vi "HEWH Determine Intellifaucet Setting.vi"(8 "Error In":errorcluster, 10 "GPM Target":dbl, 11 "Calc and Calibration":T1) -> (0 "Error Out":errorcluster, 3 "Valve % Open":dbl)   [LabVIEW 2023]
uses:
  Type Definitions/HEWH Calc and Calibration.ctl
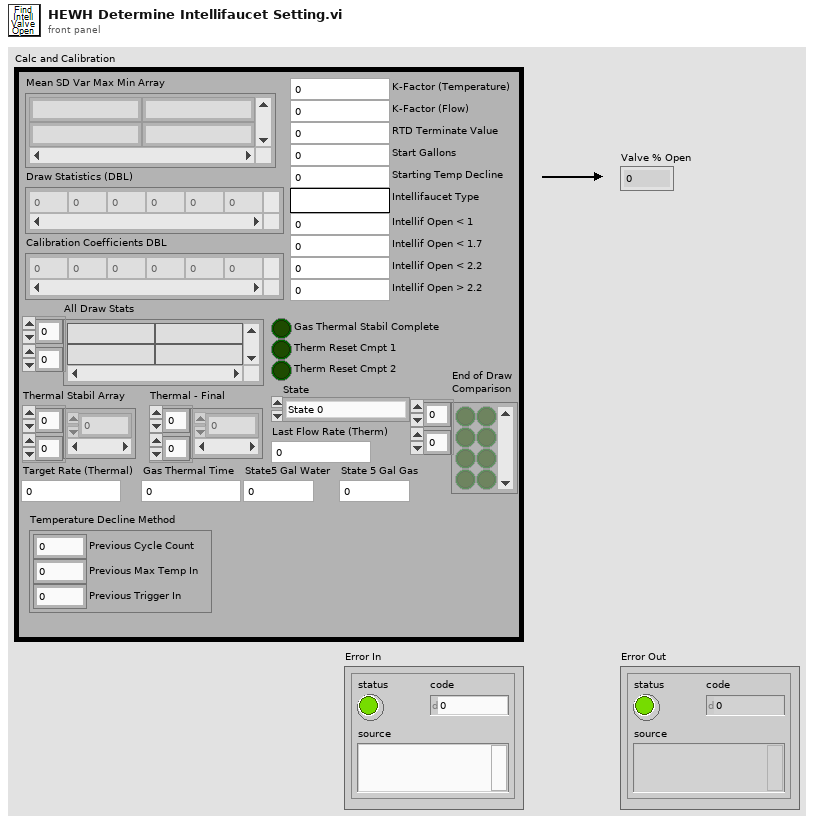
[diagram p1: front panel]
types:
  T1 = typedef "HEWH Calc and Calibration.ctl" = cluster{"Mean SD Var Max Min Array":string[][], "Draw Statistics (DBL)":dbl[][], "Calibration Coefficients DBL":dbl[][], "Start Gallons":dbl, "Starting Temp Decline":dbl, "K-Factor (Temperature)":dbl, "All Draw Stats":string[][], "RTD Terminate Value":dbl, "K-Factor (Flow)":dbl, "Intellifaucet Type":string, "Thermal Stabil Array":dbl[][], "Gas Thermal Stabil Complete":bool, "Therm Reset Cmpt 1":bool, "Therm Reset Cmpt 2":bool, "Last Flow Rate (Therm)":dbl, "State":enum16{"State 0", "State 1", "State 2", "State 3", "State 4", "State 5", "State 6"}, "Gas Thermal Time":dbl, "Target Rate (Thermal)":dbl, "Thermal - Final":dbl[][], "State5 Gal Water":dbl, "State 5 Gal Gas":dbl, "Intellif Open < 1":dbl, "Intellif Open < 1.7":dbl, "Intellif Open < 2.2":dbl, "Intellif Open > 2.2":dbl, "End of Draw\nComparison":bool[][], "Temperature Decline Method":cluster{"Previous Cycle Count":i32, "Previous Max Temp In":dbl, "Previous Trigger In":u8}}
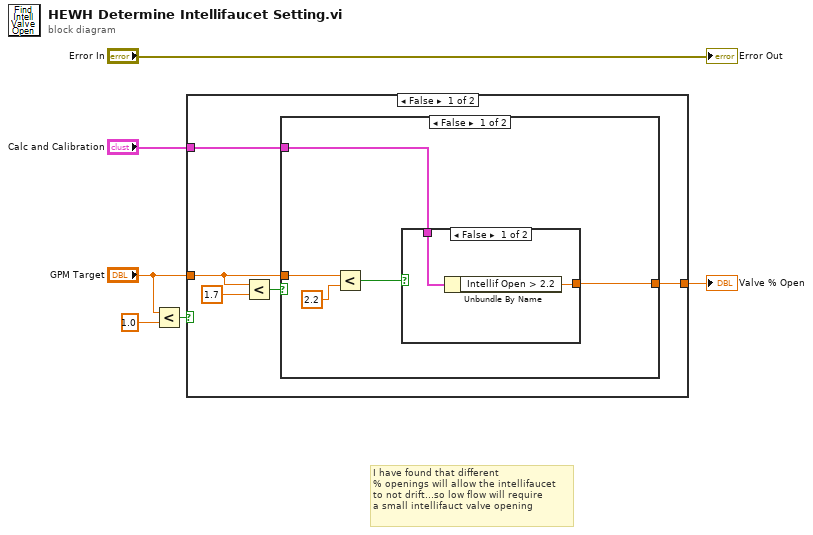
[diagram p0: block diagram]
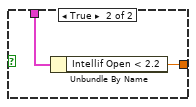
[diagram p2: hidden frame]
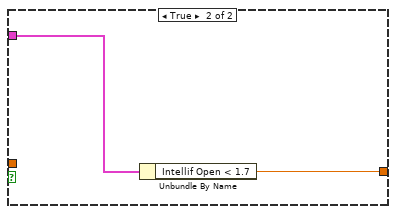
[diagram p3: hidden frame]
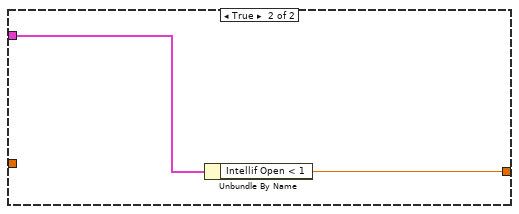
[diagram p4: hidden frame]
diagram:
  # "I have found that different\n% openings will allow the intellifaucet\nto not drift...so low flow will require\na small intellifauct valve opening"
  n1 = Less?(x="GPM Target", y=1.0) -> (x < y?=w4:bool)
  n2 = case shown="False" w4 {
    tunnel: "GPM Target" -> [w11 _]
    tunnel: [w8 w23] -> w6
    tunnel: "Calc and Calibration" -> [w7 w24]
    frame False {
      n3 = Less?(x=w11, y=1.7) -> (x < y?=w10:bool)
      n4 = case shown="False" w10 {
        tunnel: [w13 w21] -> w8
        tunnel: w11 -> [w16 _]
        tunnel: w7 -> [w12 w22]
        frame False {
          n5 = Less?(x=w16, y=2.2) -> (x < y?=w14:bool)
          n6 = case shown="False" w14 {
            tunnel: [w17 w19] -> w13
            tunnel: w12 -> [w18 w20]
            frame False {
              n7 = Unbundle By Name(w18) -> ("Intellif Open > 2.2"=w17:dbl)
            }
            frame True {
              n8 = Unbundle By Name(w20) -> ("Intellif Open < 2.2"=w19:dbl)
            }
          }
        }
        frame True {
          n9 = Unbundle By Name(w22) -> ("Intellif Open < 1.7"=w21:dbl)
        }
      }
    }
    frame True {
      n10 = Unbundle By Name(w24) -> ("Intellif Open < 1"=w23:dbl)
    }
  }
  "Valve % Open" <- w6
  "Error Out" <- "Error In"
